vi "pythonOpenSessionPopUp.vi"() -> ()   [LabVIEW 2023]
uses:
  <vilib>/Utility/config.llb/NI_LVConfig.lvlib
  <vilib>/Python/Open Venv Python Session.vi
panel:
  in  "Python environnement type":T1(ring)
  in  "Python/Environnement\npath":path
  in  "Python version":string
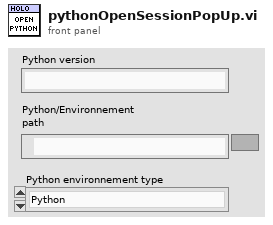
[diagram p1: front panel]
types:
  T1 = enum16{"Python", "Python virtual environnement", "Anaconda"}
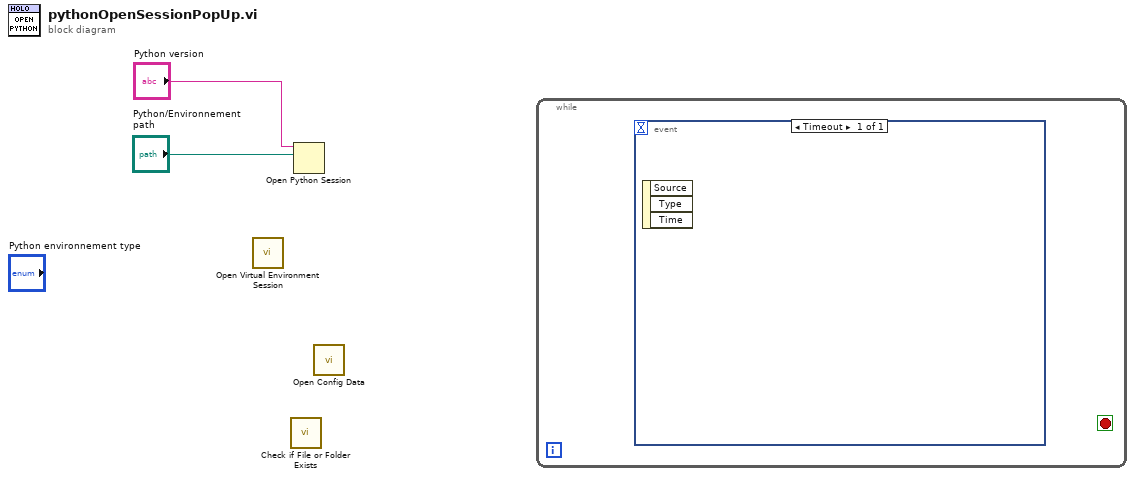
[diagram p0: block diagram]
diagram:
  n1 = call-poly <vilib>:"Open Virtual Environment Session.vi"() -> ()  [unwired: 10 in, 2 out]
  n2 = call <vilib>:"Check if File or Folder Exists.vi"() -> ()  [unwired: 9 in, 3 out]
  n3 = Open Python Session(python version="Python version", python path="Python/Environnement\npath") -> ()  [unwired: 1 in, 2 out]
  n4 = call <vilib>:"Open Config Data.vi"() -> ()  [unwired: 9 in, 3 out]
  n5 = while {
    stop <- _ stop-if-true
    n6 = event shown="[0] Timeout" {
      selector: _ -> [_]
      dyn-events: _ -> [_]
      timeout: _ -> [_]
      event Timeout {
        n7 = event-data() -> ()  [unwired: 1 in, 3 out]
      }
    }
  }
